vi "ex_4_7.vi"() -> ()   [LabVIEW 2020]
uses:
  <vilib>/numeric/Random Number (Range) U64.vi
  <vilib>/numeric/sub_Random U32.vi
panel:
  in  "stop":bool
  in  "Beginning":bool
  out "Array":i32[](array[numeric])
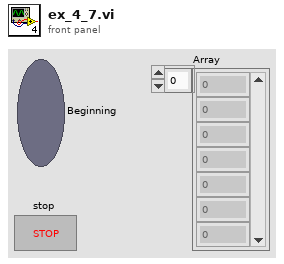
[diagram p1: front panel]
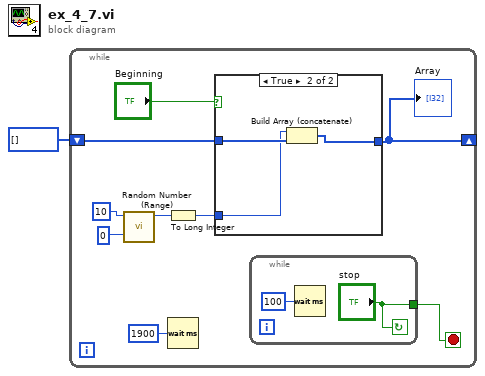
[diagram p0: block diagram]
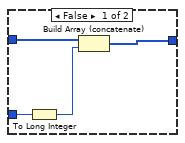
[diagram p2: hidden frame]
diagram:
  n1 = while {
    shift-right: [w6] -> _
    shift-left: i32[] [] -> [w7]
    stop <- w4 stop-if-true
    n2 = call-poly <vilib>:"Random Number (Range).vi"("lower bound (0)"=u64 0, "upper bound (100)"=u64 10) -> ("number"=w3:u64)  [unwired: 9 in]
    n3 = To Long Integer(number=w3) -> (32bit integer=w2:i32)
    n4 = Wait (ms)(milliseconds to wait=u32 1900) -> ()  [unwired: 1 out]
    n5 = case shown="True" "Beginning" {
      tunnel: w2 -> [w14 w17]
      tunnel: [w16 w18] -> w6
      tunnel: w7 -> [w15 w19]
      frame False {
        n6 = To Long Integer(number=w14) -> (32bit integer=w13:i32)
        n7 = Build Array (concatenate)(w15, w13) -> (w16:i32[])
      }
      frame True {
        n8 = Build Array (concatenate)(w17, w19) -> (w18:i32[])
      }
    }
    "Array" <- w6
    n9 = while {
      tunnel: ["stop"] -> w4
      stop <- "stop" continue-if-true
      n10 = Wait (ms)(milliseconds to wait=u32 100) -> ()  [unwired: 1 out]
    }
  }
